vi "FTW-Expression-Lexer.vi"(0 "Expression":string, 5 "Compiled Lexer Expression":i64, 7 "Lexicon":string[](array[string]), 11 "error in":errorcluster) -> (15 "error out":errorcluster)   [LabVIEW 2013]
panel:
  # "Inputs"
  # "Outputs"
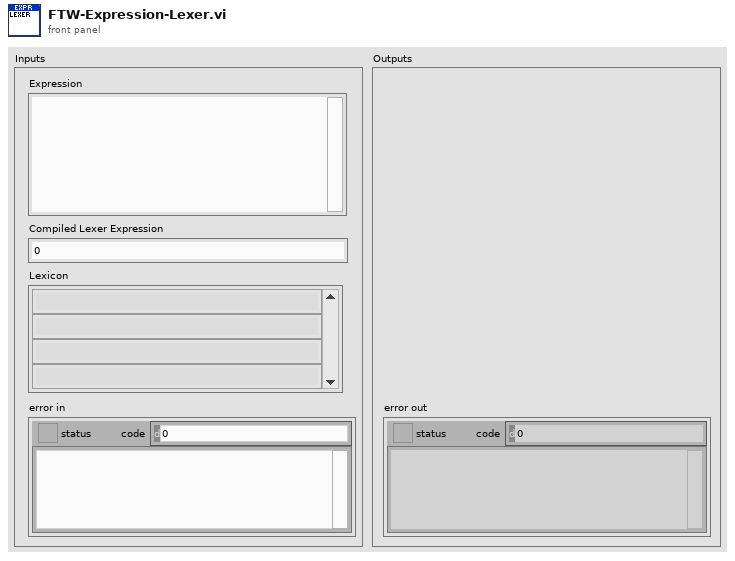
[diagram p1: front panel]
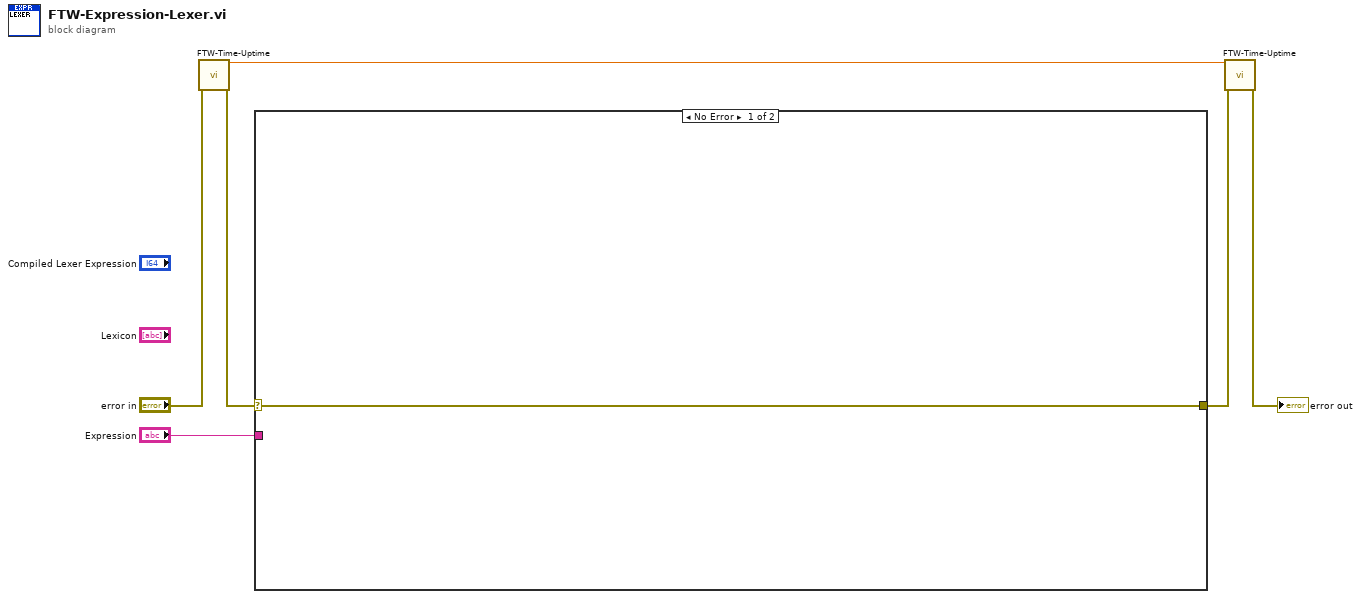
[diagram p0: block diagram]
diagram:
  n1 = call "FTW-Time-Uptime.vi"("error in"="error in") -> ("Current Uptime"=w5:dbl, "error out"=w3:errorcluster)  [unwired: 12 in, 1 out]
  n2 = case shown="No Error" w3 {
    selector: w3 -> [w7 w8]
    tunnel: [w7 w8] -> w1
    tunnel: "Expression" -> [_ _]
    frame No Error {
    }
    frame Error {
    }
  }
  n3 = call "FTW-Time-Uptime.vi"("Previous Uptime"=w5, "error in"=w1) -> ("error out"=→"error out":errorcluster)  [unwired: 11 in, 2 out]
